vi "readStatusBit.vi"(8 "error in (no error)":errorcluster, 9 "Stat Bit":T1, 10 "Status":string) -> (0 "error out":errorcluster, 2 "value":bool)   [LabVIEW 2019, in "Controller.LV.lvclass"]
uses:
  Controller.LV.lvclass
  Stat Bits--enum.ctl
  b778c5f1-1cfc-4f2b-a97f-f8a2d6e2462b.vi
  <vilib>/JDP Science/JSONtext/Find Item.vi
  <vilib>/JDP Science/JSONtext/Next JSON Value.vi
  <vilib>/JDP Science/JSONtext/String Subset.vi
  <vilib>/JDP Science/JSONtext/Parsing/Advance past next JSON Value (inlined COPY).vi
  <vilib>/JDP Science/JSONtext/Parsing/Advance past whitespace.vi
  <vilib>/JDP Science/JSONtext/Parsing/Advance past String.vi
  <vilib>/JDP Science/JSONtext/Parsing/Advance past Number.vi
  <vilib>/JDP Science/JSONtext/Parsing/Advance past Line Ending.vi
  <vilib>/JDP Science/JSONtext/Parsing/Parse Full Path or Item Name.vi
  <vilib>/JDP Science/JSONtext/Parsing/Advance past Array.vi
  <vilib>/JDP Science/JSONtext/Parsing/Advance past Object.vi
  <vilib>/JDP Science/JSONtext/support/Error Cluster From Code.vi
  <vilib>/JDP Science/JSONtext/Offset/Find Item Locations by Path.vi
  <vilib>/JDP Science/JSONtext/JSON text to Variant.vi
  <vilib>/JDP Science/JSONtext/LVClass Serializer/JSONtext LVClass Serializer.lvclass
  <vilib>/Utility/Data Type/NI_Data Type.lvlib
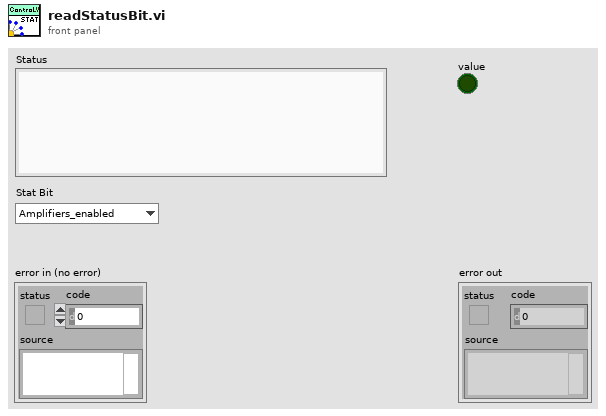
[diagram p1: front panel]
types:
  T1 = typedef "Controller.LV.lvclass/Stat Bits--enum.ctl" = enum16{"Amplifiers_enabled", "End_stop", "Thermal_protection_1", "Thermal_protection_2", "Force_zero", "Motor_on", "Closed_loop", "Encoder_at_index", "Encoder_valid", "Searching_index", "Position_reached", "Error_compensation", "Encoder_error", "Scanning", "Left_end_stop", "Right_end_stop", "Error_limit", "Searching_optimal_frequency", "Safety_timeout_triggered", "EtherCAT_acknowledge", "Emergency_stop", "Position_fail"}
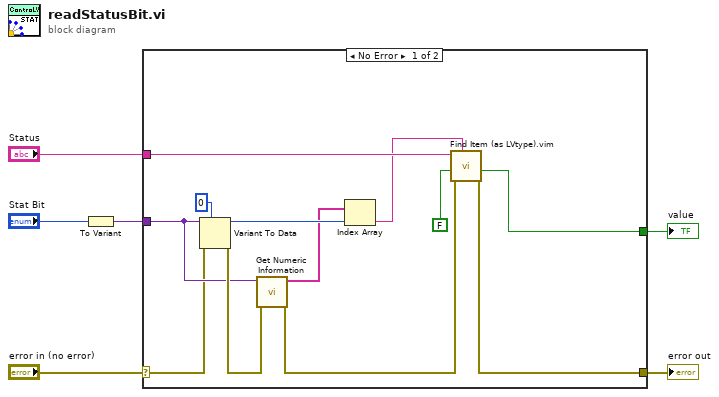
[diagram p0: block diagram]
diagram:
  n1 = To Variant(anything="Stat Bit") -> (Variant=w3:variant)
  n2 = case shown="No Error" "error in (no error)" {
    selector: "error in (no error)" -> [w13 w19]
    tunnel: [w10 w19] -> w5
    tunnel: w3 -> [w14 _]
    tunnel: "Status" -> [w8 _]
    tunnel: [w11 _] -> w1
    frame No Error {
      n3 = Variant To Data(error in=w13, type=0, Variant=w14) -> (data=w17:i32, error out=w15:errorcluster)
      n4 = call <vilib>:"Get Numeric Information.vi"("error in (no error)"=w15, "variant"=w14) -> ("error out"=w9:errorcluster, "enum names"=w16:string[])  [unwired: 6 in, 2 out]
      n5 = Index Array(array=w16, index=w17) -> (element=w7:string)
      n6 = call "Find Item (as LVtype).vim"("$Path or Item Name"=w7, "error in (no error)"=w9, "Data Type and Default Value"=FALSE, "JSON"=w8) -> ("error out"=w10:errorcluster, "Data"=w11:bool)  [unwired: 4 in, 2 out]
    }
    frame Error {
    }
  }
  "error out" <- w5
  "value" <- w1
